vi "M1M3SupportSimulatorNoGYRO.vi"   [LabVIEW 2016]
uses:
  Common_FPGA_HealthAndStatus/DataTypes/HealthAndStatusSettings.ctl
  Common_FPGA_Timestamp/DataTypes/TimestampSettings.ctl
  Common_FPGA_HealthAndStatus/DataTypes/HealthAndStatusFIFOCopySettings.ctl
  Common_FPGA_Modbus/DataTypes/ModbusPortSettings.ctl
  FPGAMockHPILC/DataTypes/MockHPILCSettings.ctl
  FPGAMockInclin/DataTypes/MockInclinSettings.ctl
  FPGAMockDisplace/DataTypes/MockDisplaceSettings.ctl
  FPGAMockFAILC/DataTypes/MockFAILCSettings.ctl
  FPGAMockAccel/DataTypes/MockAccelSettings.ctl
  FPGAMockDigitalInput/DataTypes/MockDigitalInputSettings.ctl
  <vilib>/rvi/Emulation/niFpgaGetClockAttributes.vi
  <vilib>/rvi/Emulation/niFpgaSctlEmulationGetInTimedLoop.vi
  <vilib>/rvi/Emulation/niFpgaEmulationReportErrorSimple.vi
  <vilib>/rvi/eio/common/nirviEmuTemplateMethod_errors.vi
  <vilib>/rvi/Emulation/niFpgaCriticalErrorInLSC.vi
  <vilib>/rvi/Emulation/niFpgaEmulationIsFPGAContextNoSignature.vi
  <vilib>/rvi/errors/niFpgaSetErrorForExecOnDevCompSimple.vi
  <vilib>/rvi/eio/common/nirviEmuReportErrorAndStop.vi
  <vilib>/rvi/DataTransferAndStorage/Container/Common/niFpgaContainerGetUniqueNameForEmu.vi
  <vilib>/rvi/FIFO/Fifo_Resource/nirvififoEmulationSetSize.vi
  <vilib>/rvi/FIFO/Fifo_Resource/nirviFifoEmulationQueueMgr.vi
  <instcachedir>/0/nirviFifoEmulationQueueMgr_E5CAEC123FF24DC58D834DCA3CDAA9B5.lvgen/nirviFifoEmulationQueueMgr_E5CAEC123FF24DC58D834DCA3CDAA9B5_007.vi
  <vilib>/Utility/error.llb/Clear Errors.vi
  <vilib>/rvi/FIFO/Fifo_Resource/nirvififoEmulationCreateLock.vi
  <vilib>/rvi/Emulation/niFpgaProcessEmulError.vi
  <vilib>/rvi/FIFO/Fifo_Resource/nirvififoEmulationObtainLock.vi
  <vilib>/rvi/FIFO/Fifo_Resource/nirvififoEmulationReleaseLock.vi
  <vilib>/rvi/occurrence/nirviWaitOnOccurrenceBase.vi
  <vilib>/rvi/errors/nirviReportUnexpectedCaseInternalError.vi
  <vilib>/rvi/errors/nirviReportUnexpectedCaseInternalError (U32).vi
  <vilib>/rvi/FIFO/Fifo_Resource/nirvififoEmulationDetermineInputValidOut.vi
  <instcachedir>/0/nirviFifoEmulationQueueMgr_E5CAEC123FF24DC58D834DCA3CDAA9B5.lvgen/nirviFifoEmulationQueueMgr_E5CAEC123FF24DC58D834DCA3CDAA9B5_004.vi
  <vilib>/eio/EIOMethodNode/EIOMethodNode.xnode
  <vilib>/rvi/DataTransferAndStorage/Container/XNode/niFpgaContainer.xnode
  <vilib>/rvi/FIFO/Fifo_Resource/nirvififoEmulationRead.vi
  <vilib>/rvi/FIFO/Fifo_Resource/nirvififoEmulationWrite.vi
  Common_FPGA_HealthAndStatus/FPGAHealthAndStatus.lvlib
  Common_FPGA_Timestamp/FPGATimestamp.lvlib
  Common_FPGA_Modbus/FPGAModbus.lvlib
  FPGAMockHPILC/FPGAMockHPILC.lvlib
  FPGAMockInclin/FPGAMockInclin.lvlib
  FPGAMockDisplace/FPGAMockDisplace.lvlib
  FPGAMockFAILC/FPGAMockFAILC.lvlib
  FPGAMockAccel/FPGAMockAccel.lvlib
  FPGAMockDigitalInput/FPGAMockDigitalInput.lvlib
  FPGAMockDigitalOutput/FPGAMockDigitalOutput.lvlib
types:
  T1 = typedef "FPGAMockDigitalInput.lvlib/MockDigitalInputSettings.ctl" = cluster{"BufferUpdateFIFO":refnum<k21>}
  T2 = typedef "FPGAMockAccel.lvlib/MockAccelSettings.ctl" = cluster{"BufferUpdateFIFO":refnum<k21>}
  T3 = typedef "FPGAMockFAILC.lvlib/MockFAILCSettings.ctl" = cluster{"ModbusRxDataFIFO":refnum<k21>, "ModbusTxDataFIFO":refnum<k21>, "BufferUpdateFIFO":refnum<k21>, "Code17Memory":refnum<k21>, "Code18Memory":refnum<k21>, "Code65Memory":refnum<k21>, "Code72Memory":refnum<k21>, "Code74Memory":refnum<k21>, "Code75Memory":refnum<k21>, "Code76Memory":refnum<k21>, "Code80Memory":refnum<k21>, "Code110Memory":refnum<k21>, "Code120Memory":refnum<k21>, "Code121Memory":refnum<k21>, "CRCDataFIFO":refnum<k21>, "CRCCalculateFIFO":refnum<k21>, "CRCFIFO":refnum<k21>, "Code119Memory":refnum<k21>}
  T4 = typedef "FPGAMockDisplace.lvlib/MockDisplaceSettings.ctl" = cluster{"BufferUpdateFIFO":refnum<k21>, "DisplaceMeasurementMemory":refnum<k21>}
  T5 = typedef "FPGAMockInclin.lvlib/MockInclinSettings.ctl" = cluster{"ModbusRxDataFIFO":refnum<k21>, "ModbusTxDataFIFO":refnum<k21>, "BufferUpdateFIFO":refnum<k21>, "InclinAngleMemory":refnum<k21>}
  T6 = typedef "FPGAHealthAndStatus.lvlib/HealthAndStatusFIFOCopySettings.ctl" = cluster{"InternalHealthAndStatusFIFO":refnum<k21>, "SourceHealthAndStatusFIFO":refnum<k21>}
  T7 = typedef "FPGAModbus.lvlib/ModbusPortSettings.ctl" = cluster{"TxPort":refnum<k21>, "TxDataFIFO":refnum<k21>, "TxInternalDataFIFO":refnum<k21>, "TxHealthAndStatusFIFO":refnum<k21>, "RxPort":refnum<k21>, "RxDataFIFO":refnum<k21>, "RxHealthAndStatusFIFO":refnum<k21>, "WaitForRxFrameRegister":refnum<k21>, "BaseHealthAndStatusAddress":u32, "IRQAddress":u8, "TriggerIRQRegister":refnum<k21>, "SoftwareControlledTrigger":refnum<k21>, "TimestampRegister":refnum<k21>, "TxTimestampFIFO":refnum<k21>}
  T8 = typedef "FPGAMockHPILC.lvlib/MockHPILCSettings.ctl" = cluster{"ModbusRxDataFIFO":refnum<k21>, "ModbusTxDataFIFO":refnum<k21>, "BufferUpdateFIFO":refnum<k21>, "Code17Memory":refnum<k21>, "Code18Memory":refnum<k21>, "Code65Memory":refnum<k21>, "Code66Memory":refnum<k21>, "Code67Memory":refnum<k21>, "Code72Memory":refnum<k21>, "Code80Memory":refnum<k21>, "Code110Memory":refnum<k21>, "CRCDataFIFO":refnum<k21>, "CRCCalculateFIFO":refnum<k21>, "CRCFIFO":refnum<k21>, "Code119Memory":refnum<k21>, "Code120Memory":refnum<k21>, "Code121Memory":refnum<k21>, "Code122Memory":refnum<k21>}
  T9 = typedef "FPGATimestamp.lvlib/TimestampSettings.ctl" = cluster{"TimeSource":refnum<k21>, "TimeRegister":refnum<k21>, "IterationsPerMicrosecond":i16, "UpdateFIFO":refnum<k21>, "HealthAndStatusFIFO":refnum<k21>, "HealthAndStatusAddress":i16, "IterationsPerHealthAndStatusUpdate":i16}
  T10 = typedef "FPGAHealthAndStatus.lvlib/HealthAndStatusSettings.ctl" = cluster{"InternalHealthAndStatusFIFO":refnum<k21>, "HealthAndStatusQueryFIFO":refnum<k21>, "HealthAndStatusResponseFIFO":refnum<k21>, "HealthAndStatusMemory":refnum<k21>, "MemorySize":i32}
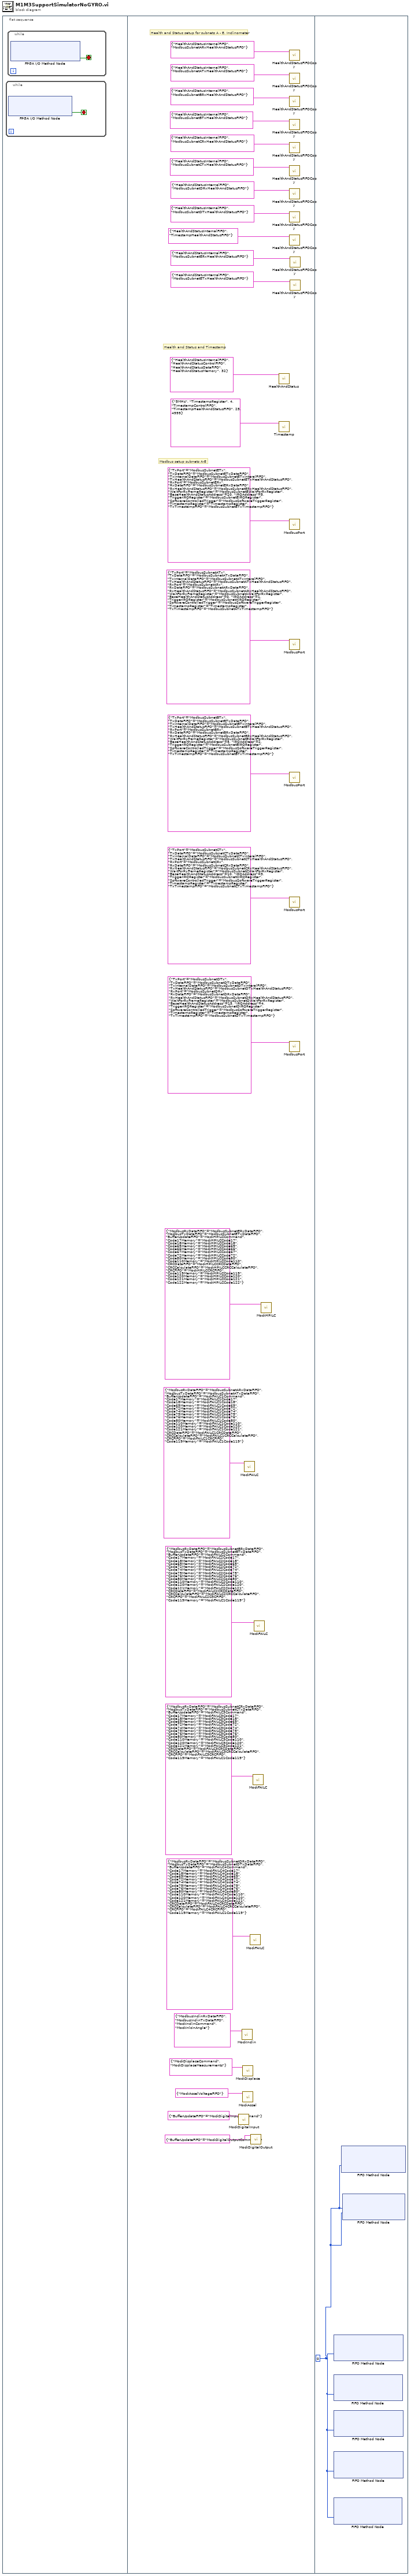
[diagram p0: block diagram]
diagram:
  n1 = flat-sequence {
    frame #0 {
      n2 = while {
        stop <- w2 stop-if-true
        n3 = xnode "FPGA I/O Method Node"() -> ("Ready"=w2:bool)  [unwired: 1 in, 1 out]
      }
      n4 = while {
        stop <- w1 stop-if-true
        n5 = xnode "FPGA I/O Method Node"() -> ("Ready"=w1:bool)  [unwired: 1 in, 1 out]
      }
    }
    frame #1 {
      # "Modbus setup subnets A-E"
      # "Health and Status and Timestamp"
      # "Health and Status setup for subnets A - E, Inclinometer"
      n6 = call "MockDigitalInput.vi"("MockDigitalInput"=T1 {"BufferUpdateFIFO"="MockDigitalInputCommand"}) -> ()  [unwired: 11 in]
      n7 = call "MockInclin.vi"("MockInclinSettings"=T5 {"ModbusRxDataFIFO"="ModbusInclinRxDataFIFO", "ModbusTxDataFIFO"="ModbusInclinTxDataFIFO", "BufferUpdateFIFO"="MockInclinCommand", "InclinAngleMemory"="MockInlcinAngle"}) -> ()  [unwired: 11 in]
      n8 = call "MockDisplace.vi"("MockDisplaceSettings"=T4 {"BufferUpdateFIFO"="MockDisplaceCommand", "DisplaceMeasurementMemory"="MockDisplaceMeasurements"}) -> ()  [unwired: 11 in]
      n9 = call "MockAccel.vi"("MockAccelSettings"=T2 {"BufferUpdateFIFO"="MockAccelVoltageFIFO"}) -> ()  [unwired: 11 in]
      n10 = call "MockFAILC.vi"("MockFAILCSettings"=T3 {"ModbusRxDataFIFO"="ModbusSubnetARxDataFIFO", "ModbusTxDataFIFO"="ModbusSubnetATxDataFIFO", "BufferUpdateFIFO"="MockFAILC1Command", "Code17Memory"="MockFAILC1Code17", "Code18Memory"="MockFAILC1Code18", "Code65Memory"="MockFAILC1Code65", "Code72Memory"="MockFAILC1Code72", "Code74Memory"="MockFAILC1Code74", "Code75Memory"="MockFAILC1Code75", "Code76Memory"="MockFAILC1Code76", "Code80Memory"="MockFAILC1Code80", "Code110Memory"="MockFAILC1Code110", "Code120Memory"="MockFAILC1Code120", "Code121Memory"="MockFAILC1Code121", "CRCDataFIFO"="MockFAILC1CRCDataFIFO", "CRCCalculateFIFO"="MockFAILC1CRCCalculateFIFO", "CRCFIFO"="MockFAILC1CRCFIFO", "Code119Memory"="MockFAILC1Code119"}) -> ()  [unwired: 11 in]
      n11 = call "MockFAILC.vi"("MockFAILCSettings"=T3 {"ModbusRxDataFIFO"="ModbusSubnetDRxDataFIFO", "ModbusTxDataFIFO"="ModbusSubnetDTxDataFIFO", "BufferUpdateFIFO"="MockFAILC4Command", "Code17Memory"="MockFAILC4Code17", "Code18Memory"="MockFAILC4Code18", "Code65Memory"="MockFAILC4Code65", "Code72Memory"="MockFAILC4Code72", "Code74Memory"="MockFAILC4Code74", "Code75Memory"="MockFAILC4Code75", "Code76Memory"="MockFAILC4Code76", "Code80Memory"="MockFAILC4Code80", "Code110Memory"="MockFAILC4Code110", "Code120Memory"="MockFAILC4Code120", "Code121Memory"="MockFAILC4Code121", "CRCDataFIFO"="MockFAILC4CRCDataFIFO", "CRCCalculateFIFO"="MockFAILC4CRCCalculateFIFO", "CRCFIFO"="MockFAILC4CRCFIFO", "Code119Memory"="MockFAILC1Code119"}) -> ()  [unwired: 11 in]
      n12 = call "MockDigitalOutput.vi"("MockDigitalOutput"=cluster{"BufferUpdateFIFO":refnum<k21>} {"BufferUpdateFIFO"="MockDigitalOutputCommand"}) -> ()  [unwired: 11 in]
      n13 = call "MockFAILC.vi"("MockFAILCSettings"=T3 {"ModbusRxDataFIFO"="ModbusSubnetCRxDataFIFO", "ModbusTxDataFIFO"="ModbusSubnetCTxDataFIFO", "BufferUpdateFIFO"="MockFAILC3Command", "Code17Memory"="MockFAILC3Code17", "Code18Memory"="MockFAILC3Code18", "Code65Memory"="MockFAILC3Code65", "Code72Memory"="MockFAILC3Code72", "Code74Memory"="MockFAILC3Code74", "Code75Memory"="MockFAILC3Code75", "Code76Memory"="MockFAILC3Code76", "Code80Memory"="MockFAILC3Code80", "Code110Memory"="MockFAILC3Code110", "Code120Memory"="MockFAILC3Code120", "Code121Memory"="MockFAILC3Code121", "CRCDataFIFO"="MockFAILC3CRCDataFIFO", "CRCCalculateFIFO"="MockFAILC3CRCCalculateFIFO", "CRCFIFO"="MockFAILC3CRCFIFO", "Code119Memory"="MockFAILC1Code119"}) -> ()  [unwired: 11 in]
      n14 = call "MockFAILC.vi"("MockFAILCSettings"=T3 {"ModbusRxDataFIFO"="ModbusSubnetBRxDataFIFO", "ModbusTxDataFIFO"="ModbusSubnetBTxDataFIFO", "BufferUpdateFIFO"="MockFAILC2Command", "Code17Memory"="MockFAILC2Code17", "Code18Memory"="MockFAILC2Code18", "Code65Memory"="MockFAILC2Code65", "Code72Memory"="MockFAILC2Code72", "Code74Memory"="MockFAILC2Code74", "Code75Memory"="MockFAILC2Code75", "Code76Memory"="MockFAILC2Code76", "Code80Memory"="MockFAILC2Code80", "Code110Memory"="MockFAILC2Code110", "Code120Memory"="MockFAILC2Code120", "Code121Memory"="MockFAILC2Code121", "CRCDataFIFO"="MockFAILC2CRCDataFIFO", "CRCCalculateFIFO"="MockFAILC2CRCCalculateFIFO", "CRCFIFO"="MockFAILC2CRCFIFO", "Code119Memory"="MockFAILC1Code119"}) -> ()  [unwired: 11 in]
      n15 = call "MockHPILC.vi"("MockHPILCSettings"=T8 {"ModbusRxDataFIFO"="ModbusSubnetERxDataFIFO", "ModbusTxDataFIFO"="ModbusSubnetETxDataFIFO", "BufferUpdateFIFO"="MockHPILCCommand", "Code17Memory"="MockHPILCCode17", "Code18Memory"="MockHPILCCode18", "Code65Memory"="MockHPILCCode65", "Code66Memory"="MockHPILCCode66", "Code67Memory"="MockHPILCCode67", "Code72Memory"="MockHPILCCode72", "Code80Memory"="MockHPILCCode80", "Code110Memory"="MockHPILCCode110", "CRCDataFIFO"="MockHPILCCRCDataFIFO", "CRCCalculateFIFO"="MockHPILCCRCCalculateFIFO", "CRCFIFO"="MockHPILCCRCFIFO", "Code119Memory"="MockHPILCCode119", "Code120Memory"="MockHPILCCode120", "Code121Memory"="MockHPILCCode121", "Code122Memory"="MockHPILCCode122"}) -> ()  [unwired: 11 in]
      n16 = call "HealthAndStatus.vi"("HealthAndStatusSettings"=T10 {"InternalHealthAndStatusFIFO"="HealthAndStatusInternalFIFO", "HealthAndStatusQueryFIFO"="HealthAndStatusControlFIFO", "HealthAndStatusResponseFIFO"="HealthAndStatusDataFIFO", "HealthAndStatusMemory"="HealthAndStatusMemory", "MemorySize"=32}) -> ()  [unwired: 11 in]
      n17 = call "Timestamp.vi"("TimestampSettings"=T9 {"TimeSource"="5MHz", "TimeRegister"="TimestampRegister", "IterationsPerMicrosecond"=4, "UpdateFIFO"="TimestampControlFIFO", "HealthAndStatusFIFO"="TimestampHealthAndStatusFIFO", "HealthAndStatusAddress"=25, "IterationsPerHealthAndStatusUpdate"=4999}) -> ()  [unwired: 11 in]
      n18 = call "HealthAndStatusFIFOCopy.vi"("HealthAndStatusSettingsFIFOCopySettings"=T6 {"InternalHealthAndStatusFIFO"="HealthAndStatusInternalFIFO", "SourceHealthAndStatusFIFO"="ModbusSubnetARxHealthAndStatusFIFO"}) -> ()  [unwired: 11 in]
      n19 = call "HealthAndStatusFIFOCopy.vi"("HealthAndStatusSettingsFIFOCopySettings"=T6 {"InternalHealthAndStatusFIFO"="HealthAndStatusInternalFIFO", "SourceHealthAndStatusFIFO"="ModbusSubnetATxHealthAndStatusFIFO"}) -> ()  [unwired: 11 in]
      n20 = call "HealthAndStatusFIFOCopy.vi"("HealthAndStatusSettingsFIFOCopySettings"=T6 {"InternalHealthAndStatusFIFO"="HealthAndStatusInternalFIFO", "SourceHealthAndStatusFIFO"="ModbusSubnetBRxHealthAndStatusFIFO"}) -> ()  [unwired: 11 in]
      n21 = call "HealthAndStatusFIFOCopy.vi"("HealthAndStatusSettingsFIFOCopySettings"=T6 {"InternalHealthAndStatusFIFO"="HealthAndStatusInternalFIFO", "SourceHealthAndStatusFIFO"="ModbusSubnetBTxHealthAndStatusFIFO"}) -> ()  [unwired: 11 in]
      n22 = call "HealthAndStatusFIFOCopy.vi"("HealthAndStatusSettingsFIFOCopySettings"=T6 {"InternalHealthAndStatusFIFO"="HealthAndStatusInternalFIFO", "SourceHealthAndStatusFIFO"="ModbusSubnetCRxHealthAndStatusFIFO"}) -> ()  [unwired: 11 in]
      n23 = call "HealthAndStatusFIFOCopy.vi"("HealthAndStatusSettingsFIFOCopySettings"=T6 {"InternalHealthAndStatusFIFO"="HealthAndStatusInternalFIFO", "SourceHealthAndStatusFIFO"="ModbusSubnetCTxHealthAndStatusFIFO"}) -> ()  [unwired: 11 in]
      n24 = call "HealthAndStatusFIFOCopy.vi"("HealthAndStatusSettingsFIFOCopySettings"=T6 {"InternalHealthAndStatusFIFO"="HealthAndStatusInternalFIFO", "SourceHealthAndStatusFIFO"="ModbusSubnetDRxHealthAndStatusFIFO"}) -> ()  [unwired: 11 in]
      n25 = call "HealthAndStatusFIFOCopy.vi"("HealthAndStatusSettingsFIFOCopySettings"=T6 {"InternalHealthAndStatusFIFO"="HealthAndStatusInternalFIFO", "SourceHealthAndStatusFIFO"="ModbusSubnetDTxHealthAndStatusFIFO"}) -> ()  [unwired: 11 in]
      n26 = call "HealthAndStatusFIFOCopy.vi"("HealthAndStatusSettingsFIFOCopySettings"=T6 {"InternalHealthAndStatusFIFO"="HealthAndStatusInternalFIFO", "SourceHealthAndStatusFIFO"="TimestampHealthAndStatusFIFO"}) -> ()  [unwired: 11 in]
      n27 = call "ModbusPort.vi"("ModbusPortSettings"=T7 {"TxPort"="ModbusSubnetETx", "TxDataFIFO"="ModbusSubnetETxDataFIFO", "TxInternalDataFIFO"="ModbusSubnetETxInteralFIFO", "TxHealthAndStatusFIFO"="ModbusSubnetETxHealthAndStatusFIFO", "RxPort"="ModbusSubnetERx", "RxDataFIFO"="ModbusSubnetERxDataFIFO", "RxHealthAndStatusFIFO"="ModbusSubnetERxHealthAndStatusFIFO", "WaitForRxFrameRegister"="ModbusSubnetEWaitForRxRegister", "BaseHealthAndStatusAddress"=20, "IRQAddress"=5, "TriggerIRQRegister"="ModbusSubnetEIRQRegister", "SoftwareControlledTrigger"="ModbusSoftwareTriggerRegister", "TimestampRegister"="TimestampRegister", "TxTimestampFIFO"="ModbusSubnetETxTimestampFIFO"}) -> ()  [unwired: 10 in]
      n28 = call "ModbusPort.vi"("ModbusPortSettings"=T7 {"TxPort"="ModbusSubnetATx", "TxDataFIFO"="ModbusSubnetATxDataFIFO", "TxInternalDataFIFO"="ModbusSubnetATxInteralFIFO", "TxHealthAndStatusFIFO"="ModbusSubnetATxHealthAndStatusFIFO", "RxPort"="ModbusSubnetARx", "RxDataFIFO"="ModbusSubnetARxDataFIFO", "RxHealthAndStatusFIFO"="ModbusSubnetARxHealthAndStatusFIFO", "WaitForRxFrameRegister"="ModbusSubnetAWaitForRxRegister", "BaseHealthAndStatusAddress"=0, "IRQAddress"=1, "TriggerIRQRegister"="ModbusSubnetAIRQRegister", "SoftwareControlledTrigger"="ModbusSoftwareTriggerRegister", "TimestampRegister"="TimestampRegister", "TxTimestampFIFO"="ModbusSubnetATxTimestampFIFO"}) -> ()  [unwired: 10 in]
      n29 = call "ModbusPort.vi"("ModbusPortSettings"=T7 {"TxPort"="ModbusSubnetBTx", "TxDataFIFO"="ModbusSubnetBTxDataFIFO", "TxInternalDataFIFO"="ModbusSubnetBTxInteralFIFO", "TxHealthAndStatusFIFO"="ModbusSubnetBTxHealthAndStatusFIFO", "RxPort"="ModbusSubnetBRx", "RxDataFIFO"="ModbusSubnetBRxDataFIFO", "RxHealthAndStatusFIFO"="ModbusSubnetBRxHealthAndStatusFIFO", "WaitForRxFrameRegister"="ModbusSubnetBWaitForRxRegister", "BaseHealthAndStatusAddress"=5, "IRQAddress"=2, "TriggerIRQRegister"="ModbusSubnetBIRQRegister", "SoftwareControlledTrigger"="ModbusSoftwareTriggerRegister", "TimestampRegister"="TimestampRegister", "TxTimestampFIFO"="ModbusSubnetBTxTimestampFIFO"}) -> ()  [unwired: 10 in]
      n30 = call "ModbusPort.vi"("ModbusPortSettings"=T7 {"TxPort"="ModbusSubnetCTx", "TxDataFIFO"="ModbusSubnetCTxDataFIFO", "TxInternalDataFIFO"="ModbusSubnetCTxInteralFIFO", "TxHealthAndStatusFIFO"="ModbusSubnetCTxHealthAndStatusFIFO", "RxPort"="ModbusSubnetCRx", "RxDataFIFO"="ModbusSubnetCRxDataFIFO", "RxHealthAndStatusFIFO"="ModbusSubnetCRxHealthAndStatusFIFO", "WaitForRxFrameRegister"="ModbusSubnetCWaitForRxRegister", "BaseHealthAndStatusAddress"=10, "IRQAddress"=3, "TriggerIRQRegister"="ModbusSubnetCIRQRegister", "SoftwareControlledTrigger"="ModbusSoftwareTriggerRegister", "TimestampRegister"="TimestampRegister", "TxTimestampFIFO"="ModbusSubnetCTxTimestampFIFO"}) -> ()  [unwired: 10 in]
      n31 = call "ModbusPort.vi"("ModbusPortSettings"=T7 {"TxPort"="ModbusSubnetDTx", "TxDataFIFO"="ModbusSubnetDTxDataFIFO", "TxInternalDataFIFO"="ModbusSubnetDTxInteralFIFO", "TxHealthAndStatusFIFO"="ModbusSubnetDTxHealthAndStatusFIFO", "RxPort"="ModbusSubnetDRx", "RxDataFIFO"="ModbusSubnetDRxDataFIFO", "RxHealthAndStatusFIFO"="ModbusSubnetDRxHealthAndStatusFIFO", "WaitForRxFrameRegister"="ModbusSubnetDWaitForRxRegister", "BaseHealthAndStatusAddress"=15, "IRQAddress"=4, "TriggerIRQRegister"="ModbusSubnetDIRQRegister", "SoftwareControlledTrigger"="ModbusSoftwareTriggerRegister", "TimestampRegister"="TimestampRegister", "TxTimestampFIFO"="ModbusSubnetDTxTimestampFIFO"}) -> ()  [unwired: 10 in]
      n32 = call "HealthAndStatusFIFOCopy.vi"("HealthAndStatusSettingsFIFOCopySettings"=T6 {"InternalHealthAndStatusFIFO"="HealthAndStatusInternalFIFO", "SourceHealthAndStatusFIFO"="ModbusSubnetERxHealthAndStatusFIFO"}) -> ()  [unwired: 11 in]
      n33 = call "HealthAndStatusFIFOCopy.vi"("HealthAndStatusSettingsFIFOCopySettings"=T6 {"InternalHealthAndStatusFIFO"="HealthAndStatusInternalFIFO", "SourceHealthAndStatusFIFO"="ModbusSubnetETxHealthAndStatusFIFO"}) -> ()  [unwired: 11 in]
    }
    frame #2 {
      w31 = 0 ("Timeout")
      n34 = xnode ("FIFO Method Node")("Timeout"=w31) -> ()  [unwired: 1 in, 3 out]
      n35 = xnode ("FIFO Method Node")("Timeout"=w31) -> ()  [unwired: 1 in, 3 out]
      n36 = xnode ("FIFO Method Node")("Timeout"=w31) -> ()  [unwired: 1 in, 3 out]
      n37 = xnode ("FIFO Method Node")("Timeout"=w31) -> ()  [unwired: 1 in, 3 out]
      n38 = xnode ("FIFO Method Node")("Timeout"=w31) -> ()  [unwired: 1 in, 3 out]
      n39 = xnode ("FIFO Method Node")("Timeout"=w31) -> ()  [unwired: 1 in, 3 out]
      n40 = xnode ("FIFO Method Node")("Element"=w31, "Timeout"=w31) -> ()  [unwired: 1 in, 2 out]
    }
  }
